vi "StringROItoNumROI.vi"(1 "String":string) -> (0 "Array":i32[](array[numeric]))   [LabVIEW 2011]
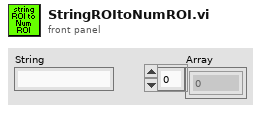
[diagram p1: front panel]
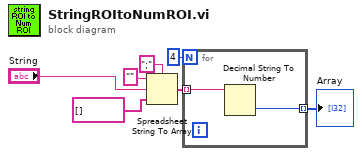
[diagram p0: block diagram]
diagram:
  n1 = Spreadsheet String To Array(delimiter (Tab)=";", format string="" ("spreadsheet string"), spreadsheet string="String", array type (2D Dbl)=string[] []) -> (array=w2:string[])
  n2 = for {
    N: 4 -> [_]
    tunnel: w2 -> [w9] mode=indexing
    tunnel: [w8] -> w6 mode=indexing
    n3 = Decimal String To Number(string=w9) -> (number=w8:i32)  [unwired: 2 in, 1 out]
  }
  "Array" <- w6
